vi "fgv_cache.vi"(4 "Initialization Count (0)":i32, 6 "Index in":i32, 7 "Operation":T1(ring)=enum."Get Cached Value", 8 "error in":errorcluster, 10 "Value in":variant, 11 "VISA resource name":refnum<visa-resource-name>) -> (0 "error out":errorcluster, 2 "Cache Value out":variant, 3 "VISA resource name out":refnum<visa-resource-name>)   [LabVIEW 2014, in "rszvl_rsidr_core.lvlib"]
uses:
  rszvl_rsidr_core.lvlib
  type_Error_Codes.ctl
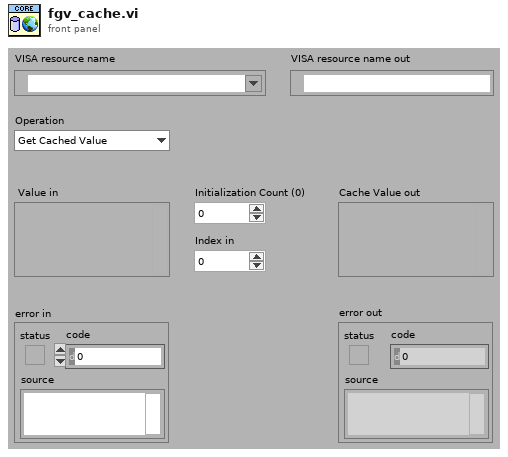
[diagram p1: front panel]
types:
  T1 = enum16{"Initialize", "Get Cached Value", "Set Cached Value", "Clear"}
  T2 = typedef "rszvl_rsidr_core.lvlib/type_Error_Codes.ctl" = enum16{"No_error", "VISA_err_ResourceNotFound", "VISA_err_Timeout", "VISA_warn_MoreDataAvailable", "RS_err_MissingCallback", "RS_err_InvalidAttribute", "RS_err_InvalidValue", "RS_err_UnknownResource", "RS_err_AlreadyInitialized", "RS_err_InstrumentStatus", "RS_err_BadRepCapName", "RS_err_TypesMismatch", "RS_err_ValueNotSupported", "RS_err_InvalidRngTable", "RS_err_IDqueryFail", "RS_err_UnexpResponse", "VISA_warn_ConfigNotLoaded", "RS_err_AttributeNotReadable", "RS_err_AttributeNotWritable", "RS_err_InstrumentType", "RS_err_InstrumentOption", "VISA_err_InvalidSize", "RS_err_ReliabilityIndicator", "VISA_warn_UnknownStatus", "VISA_warn_TermCharRead", "VISA_err_IO_error"}
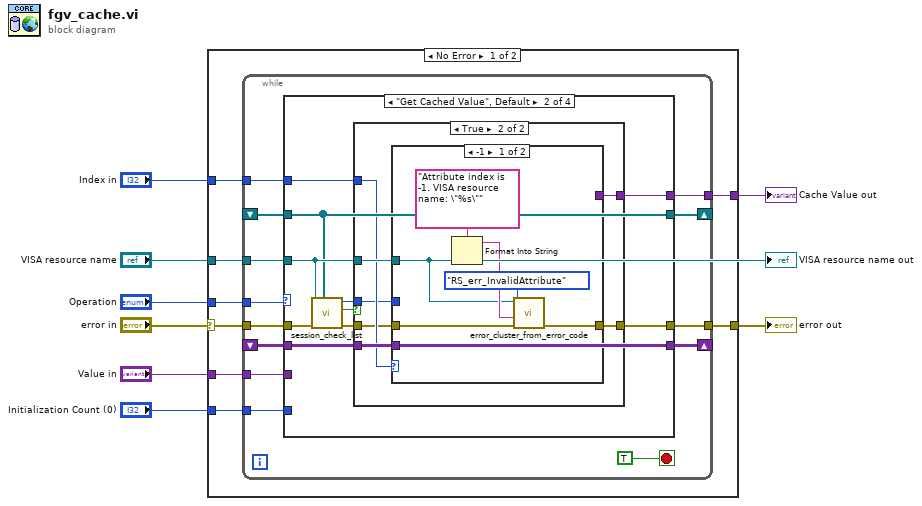
[diagram p0: block diagram]
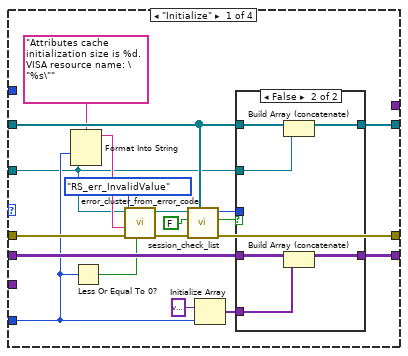
[diagram p2: hidden frame]
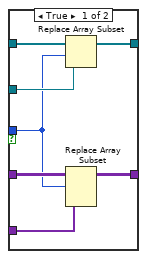
[diagram p3: hidden frame]
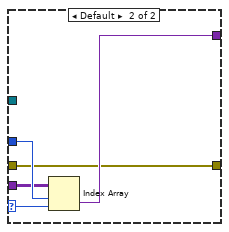
[diagram p5: hidden frame]
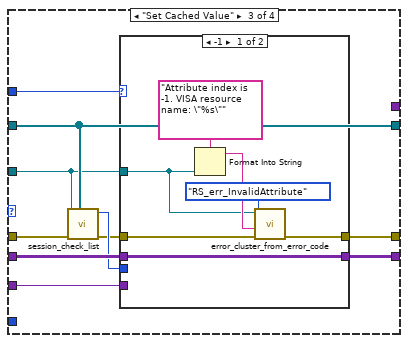
[diagram p6: hidden frame]
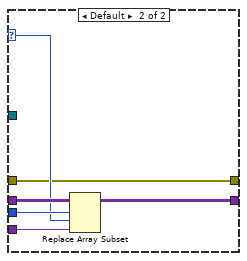
[diagram p7: hidden frame]
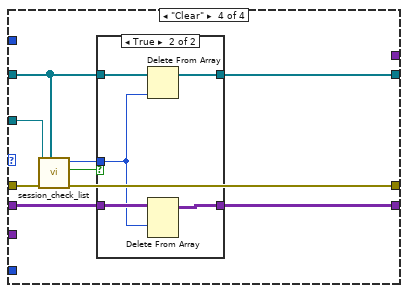
[diagram p8: hidden frame]
diagram:
  n1 = case shown="No Error" "error in" {
    selector: "error in" -> [w10 w130]
    tunnel: "Index in" -> [w16 _]
    tunnel: "VISA resource name" -> [w9 _]
    tunnel: [w11 w130] -> w7
    tunnel: [w15 _] -> w6
    tunnel: "Value in" -> [w14 _]
    tunnel: "Operation" -> [w13 _]
    tunnel: "Initialization Count (0)" -> [w12 _]
    frame No Error {
      n2 = while {
        tunnel: [w29] -> w11
        tunnel: w16 -> [w28]
        tunnel: w9 -> [w27]
        shift-right: [w24] -> _
        shift-left: _ -> [w25]
        shift-right: [w22] -> _
        shift-left: _ -> [w23]
        tunnel: [w21] -> w15
        tunnel: w14 -> [w20]
        tunnel: w13 -> [w19]
        tunnel: w12 -> [w18]
        tunnel: w10 -> [w17]
        stop <- TRUE stop-if-true
        n3 = case shown="\"Get Cached Value\", Default" w19 {
          tunnel: [w41 w70 w97 w114] -> w29
          tunnel: w28 -> [_ w71 w100 _]
          tunnel: w27 -> [w31 w66 w91 w118]
          tunnel: w25 -> [w44 w65 w94 w117]
          tunnel: [w48 w65 w94 w122] -> w24
          tunnel: w23 -> [w47 w69 w99 w121]
          tunnel: [w46 w69 w98 w120] -> w22
          tunnel: [_ w68 _ _] -> w21
          tunnel: w20 -> [_ _ w96 _]
          tunnel: w18 -> [w35 _ _ _]
          tunnel: w17 -> [w39 w67 w95 w119]
          frame "Initialize" {
            n4 = Format Into String(format string="Attributes cache initialization size is %d. VISA resource name: \"%s\"", w35, w31) -> (resulting string=w33:string)  [unwired: 2 in, 1 out]
            n5 = Less Or Equal To 0?(x=w35) -> (x <= 0?=w37:bool)
            n6 = call "error_cluster_from_error_code.vi"("error creation enabled (T)"=w37, "error in"=w39, "error message (\"\")"=w33, "Error Enum in"=type_Error_Codes."RS_err_InvalidValue", "VISA resource name"=w31) -> ("error out"=w38:errorcluster, "VISA resource name out"=w30:refnum<visa-resource-name>)  [unwired: 5 in]
            n7 = call "session_check_list.vi"("VISA resource names in"=w44, "error in"=w38, "Error if not found (T)"=FALSE, "VISA resource name"=w30) -> ("error out"=w41:errorcluster, "Found in the list"=w43:bool, "Session list index out"=w42:i32)  [unwired: 5 in]
            n8 = Initialize Array(variant ("element"), w35) -> (w45:variant[])
            n9 = case shown="False" w43 {
              tunnel: [w54 w57] -> w48
              tunnel: w44 -> [w55 w61]
              tunnel: w31 -> [w51 w59]
              tunnel: w47 -> [w53 w60]
              tunnel: w45 -> [w50 w56]
              tunnel: [w52 w58] -> w46
              tunnel: w42 -> [w49 _]
              frame True {
                n10 = Replace Array Subset(array=w55, new element=w51, index=w49) -> (w54:refnum<visa-resource-name>[])
                n11 = Replace Array Subset(array=w53, new element=w50, index (row)=w49) -> (w52:variant[][])  [unwired: 1 in]
              }
              frame False {
                n12 = Build Array (concatenate)(w61, w59) -> (w57:refnum<visa-resource-name>[])
                n13 = Build Array (concatenate)(w60, w56) -> (w58:variant[][])
              }
            }
          }
          frame "Get Cached Value", Default {
            n14 = call "session_check_list.vi"("VISA resource names in"=w65, "error in"=w67, "VISA resource name"=w66) -> ("error out"=w64:errorcluster, "Found in the list"=w62:bool, "Session list index out"=w63:i32)  [unwired: 6 in]
            n15 = case shown="True" w62 {
              tunnel: w71 -> [_ w76]
              tunnel: [w72 w78] -> w70
              tunnel: w69 -> [_ w79]
              tunnel: [_ w77] -> w68
              tunnel: w64 -> [w72 w75]
              tunnel: w66 -> [_ w73]
              tunnel: w63 -> [_ w74]
              frame False {
              }
              frame True {
                n16 = case shown="-1" w76 {
                  selector: w76 -> [_ w88]
                  tunnel: w79 -> [_ w87]
                  tunnel: w74 -> [_ w89]
                  tunnel: [w85 w86] -> w78
                  tunnel: [_ w90] -> w77
                  tunnel: w75 -> [w84 w86]
                  tunnel: w73 -> [w80 _]
                  frame -1 {
                    n17 = Format Into String(format string="Attribute index is -1. VISA resource name: \"%s\"" ("source"), w80) -> (resulting string=w82:string)  [unwired: 2 in, 1 out]
                    n18 = call "error_cluster_from_error_code.vi"("error in"=w84, "error message (\"\")"=w82, "Error Enum in"=type_Error_Codes."RS_err_InvalidAttribute", "VISA resource name"=w80) -> ("error out"=w85:errorcluster)  [unwired: 6 in, 1 out]
                  }
                  frame Default {
                    n19 = Index Array(array=w87, index (row)=w89, index (col)=w88) -> (element=w90:variant)
                  }
                }
              }
            }
          }
          frame "Set Cached Value" {
            n20 = call "session_check_list.vi"("VISA resource names in"=w94, "error in"=w95, "VISA resource name"=w91) -> ("error out"=w92:errorcluster, "Session list index out"=w93:i32)  [unwired: 6 in, 1 out]
            n21 = case shown="-1" w100 {
              selector: w100 -> [_ w110]
              tunnel: w99 -> [w107 w112]
              tunnel: [w107 w113] -> w98
              tunnel: w93 -> [_ w111]
              tunnel: [w106 w108] -> w97
              tunnel: w96 -> [_ w109]
              tunnel: w92 -> [w105 w108]
              tunnel: w91 -> [w101 _]
              frame -1 {
                n22 = Format Into String(format string="Attribute index is -1. VISA resource name: \"%s\"" ("source"), w101) -> (resulting string=w103:string)  [unwired: 2 in, 1 out]
                n23 = call "error_cluster_from_error_code.vi"("error in"=w105, "error message (\"\")"=w103, "Error Enum in"=type_Error_Codes."RS_err_InvalidAttribute", "VISA resource name"=w101) -> ("error out"=w106:errorcluster)  [unwired: 6 in, 1 out]
              }
              frame Default {
                n24 = Replace Array Subset(array=w112, new element=w109, index (row)=w111, index (col)=w110) -> (w113:variant[][])
              }
            }
          }
          frame "Clear" {
            n25 = call "session_check_list.vi"("VISA resource names in"=w117, "error in"=w119, "VISA resource name"=w118) -> ("error out"=w114:errorcluster, "Found in the list"=w116:bool, "Session list index out"=w115:i32)  [unwired: 6 in]
            n26 = case shown="True" w116 {
              tunnel: [w124 w129] -> w122
              tunnel: w121 -> [w123 w128]
              tunnel: [w123 w127] -> w120
              tunnel: w117 -> [w124 w126]
              tunnel: w115 -> [_ w125]
              frame False {
              }
              frame True {
                n27 = Delete From Array(array=w126, index=w125) -> (array with subset deleted=w129:refnum<visa-resource-name>[])  [unwired: 1 in, 1 out]
                n28 = Delete From Array(array=w128, index (row)=w125) -> (array with subset deleted=w127:variant[][])  [unwired: 2 in, 1 out]
              }
            }
          }
        }
      }
    }
    frame Error {
    }
  }
  "error out" <- w7
  "Cache Value out" <- w6
  "VISA resource name out" <- "VISA resource name"
